vi "AES ECU Event Measurement - End Angle.vi"(6 "Cycles to Filter":u16, 10 "Digital Input Pulse":bool, 11 "Crank or Cyle Angle":fxp<+,61,10>) -> (0 "End Angle (degrees)":fxp<+,61,10> format="%.55g")   [LabVIEW 2010, in "AES.lvlib" / "AES FPGA.lvlib"]
doc: "This IP inputs the fuel injector or ignition coil digital signals from an ECU and determines the End Angle of the pulses for those signals. This IP allows you to input either the crank (0-360) or cycle (0-720) angles. A \"Cycles to Filter\" input is also accepted in order to filter the digital inputs for a specified number of SCTL iterations. This is necessary since ECUs often output very noisy signals, and we need to filter it to get accurate calculations on the Start and End Angles."
uses:
  AES FPGA.lvlib
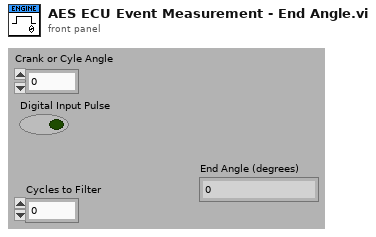
[diagram p1: front panel]
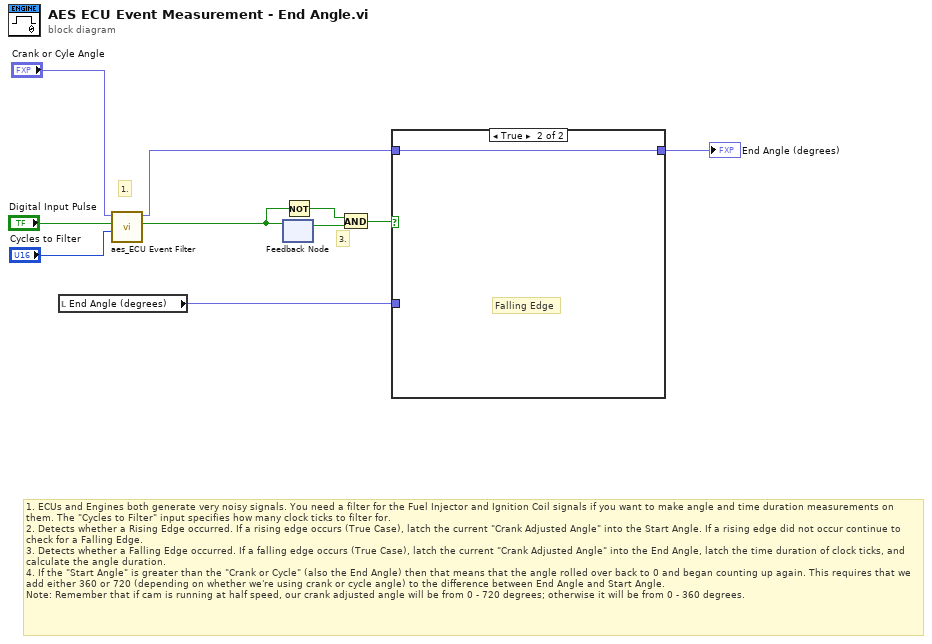
[diagram p0: block diagram]
diagram:
  # "3."
  # "1. ECUs and Engines both generate very noisy signals. You need a filter for the Fuel Injector and Ignition Coil signals if you want to make angle and time duration measurements on them. The \"Cycles to Filter\" input specifies how many clock ticks to filter for.\n2. Detects whether a Rising Edge occurred. If a rising edge occurs (True Case), latch the current \"Crank Adjusted Angle\" into the Start Angle. If a rising edge did not occur continue to check for a Falling Edge.\n3. Detects whether a Falling Edge occurred. If a falling edge occurs (True Case), latch the current \"Crank Adjusted Angle\" into the End Angle, latch the time duration of clock ticks, and calculate the angle duration.\n4. If the \"Start Angle\" is greater than the \"Crank or Cycle\" (also the End Angle) then that means that the angle rolled over back to 0 and began counting up again. This requires that we add either 360 or 720 (depending on whether we're using crank or cycle angle) to the difference between End Angle and Start Angle.\nNote: Remember that if cam is running at half speed, our crank adjusted angle will be from 0 - 720 degrees; otherwise it will be from 0 - 360 degrees."
  # "1."
  n1 = local read "End Angle (degrees)"() -> (w9:fxp<+,61,10>)
  n2 = call "aes_ECU Event Filter.vi"("Cycles to Filter"="Cycles to Filter", "Input Signal"="Digital Input Pulse", "Input Angle (degrees)"="Crank or Cyle Angle") -> ("Output Filtered Signal"=w6:bool, "Transitioned Angle"=w7:fxp<+,61,10>)  [unwired: 7 in]
  n3 = feedback #1() -> (w2:bool)  [unwired: 1 out]
  n4 = feedback-in #1(w6) -> ()
  n5 = Not(x=w6) -> (.not. x?=w1:bool)
  n6 = And(x=w1, y=w2) -> (x .and. y?=w3:bool)
  n7 = case shown="True" w3 {
    tunnel: w7 -> [_ w12]
    tunnel: [w11 w12] -> w10
    tunnel: w9 -> [w11 _]
    frame False {
    }
    frame True {
      # "Falling Edge"
    }
  }
  "End Angle (degrees)" <- w10
